vi "Close VI Ref.vi"(8 "error in (no error)":errorcluster, 11 "LUnit Test Case In":refnum<class "LUnit Test Case.lvclass">) -> (0 "error out":errorcluster, 3 "LUnit Test Case Out":refnum<class "LUnit Test Case.lvclass">)   [LabVIEW 2020, in "LUnit Test Case.lvclass"]
uses:
  LUnit Test Case.lvclass
  LUnit Test Case.lvclass/LUnit Test Case.ctl
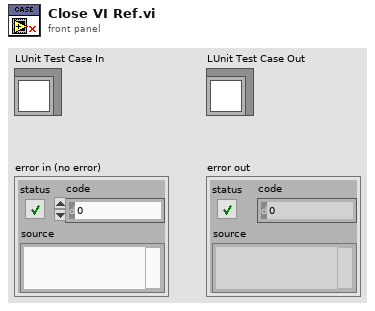
[diagram p1: front panel]
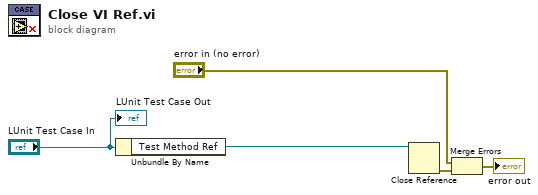
[diagram p0: block diagram]
diagram:
  n1 = Unbundle By Name("LUnit Test Case In") -> ("Test Method Ref"=w1:refnum<vi>)
  n2 = Close Reference(reference=w1) -> (error out=w5:errorcluster)  [unwired: 1 in]
  n3 = Merge Errors("error in (no error)", w5) -> (→"error out":errorcluster)
  "LUnit Test Case Out" <- "LUnit Test Case In"
